vi "MOVE BIAS.vi"(0 "SweepQ in":refnum<queue>, 1 "x":dbl, 2 "return value":cluster{"x":dbl, "y":dbl}, 5 "ScanQ in":refnum<queue>, 7 "Boolean":bool, 11 "error in (no error)":errorcluster, 12 "y":dbl, 13 "Bias in":T1 {"Final Y (m)" format="%.3p"; "Final X (m)" format="%.3p"}) -> (3 "X (m)":sgl, 4 "SweepQ out":refnum<queue>, 6 "ScanQ out":refnum<queue>, 14 "Y (m)":sgl, 15 "error out":errorcluster)   [LabVIEW 2025]
uses:
  STM-Auto-Project/QMH CTLS/Scan_Params (QMH).ctl
  STM-Auto-Project/QMH CTLS/Sweeper.ctl
  Magnetic Drift Correction/Bias Cont QMH.ctl
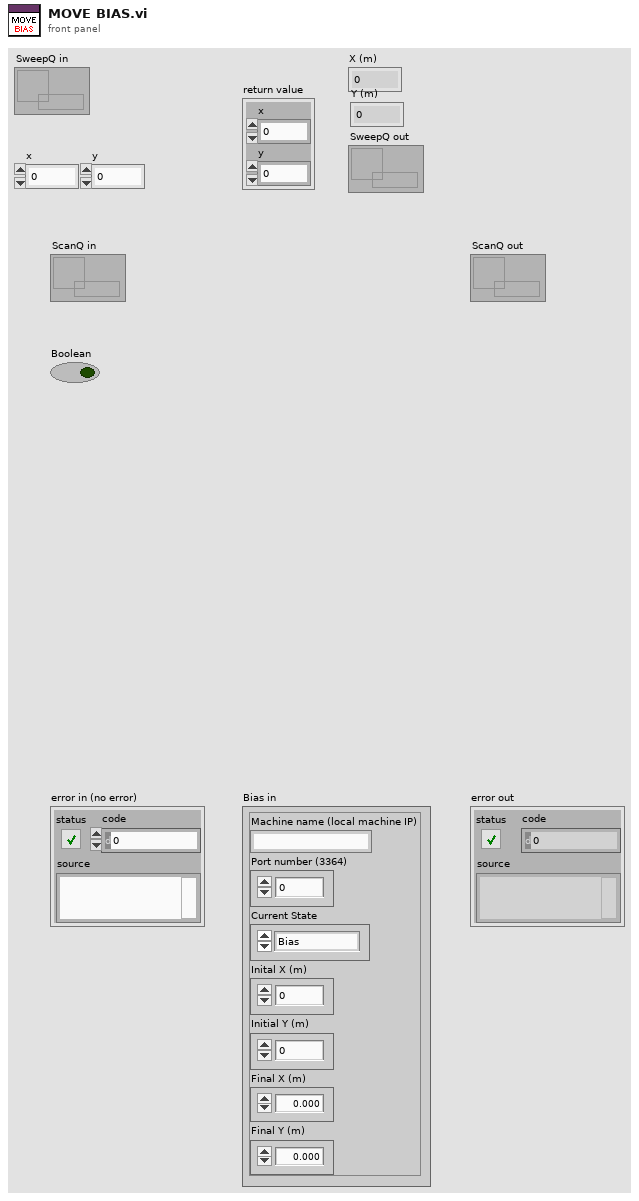
[diagram p1: front panel]
types:
  T1 = typedef "Bias Cont QMH.ctl" = cluster{"Machine name (local machine IP)":string, "Port number (3364)":u32, "Current State":enum16{"Bias", "Stop"}, "Inital X (m)":dbl, "Initial Y (m)":dbl, "Final X (m)":sgl, "Final Y (m)":sgl}
  T2 = enum16{"NO CHANGE", "SET TEMP & FIELD", "SWEEP IDLE", "NEXT TEMP & FIELD", "SWEEP DONE"}
  T3 = typedef "Sweeper.ctl" = cluster{"Temps(K)":dbl[], "Fields(T)":dbl[], "Sweep States":enum16{"NO CHANGE", "SET TEMP & FIELD", "SWEEP IDLE", "NEXT TEMP & FIELD", "SWEEP DONE"}}
  T4 = enum16{"1. BIAS", "2. INIT_SCAN", "3. SCAN_IDLE", "4. INTER_SCAN", "5. NEW_COORDS_&_FRAME", "6. FINAL_SCAN", "7. POLL BIAS ", "8. STOP"}
  T5 = typedef "Scan_Params (QMH).ctl" = cluster{"Setpoint (I)":dbl[], "Bias (V)":dbl[], "Number of scans":u8, "Port number (3364)":u32, "Avoid zero threshold (V)":dbl, "Current State":enum16{"1. BIAS", "2. INIT_SCAN", "3. SCAN_IDLE", "4. INTER_SCAN", "5. NEW_COORDS_&_FRAME", "6. FINAL_SCAN", "7. POLL BIAS ", "8. STOP"}}
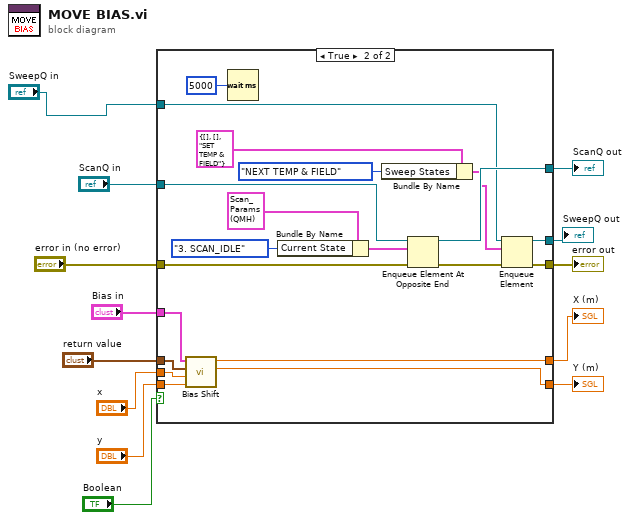
[diagram p0: block diagram]
diagram:
  n1 = case shown="True" "Boolean" {
    tunnel: "return value" -> [_ w29]
    tunnel: "ScanQ in" -> [w17 w33]
    tunnel: [w17 w34] -> w10
    tunnel: [w16 w35] -> w11
    tunnel: "error in (no error)" -> [w16 w31]
    tunnel: [_ w36] -> w2
    tunnel: [w15 w28] -> w6
    tunnel: "Bias in" -> [_ w27]
    tunnel: "SweepQ in" -> [_ w25]
    tunnel: [w14 w24] -> w5
    tunnel: "x" -> [w15 w23]
    tunnel: "y" -> [w14 w22]
    frame False {
    }
    frame True {
      n2 = call "Bias Shift.vi"("y"=w22, "x"=w23, "Translation (m)"=w29, "Bias Controller"=w27) -> ("Y (m)"=w24:sgl, "X (m)"=w28:sgl)  [unwired: 6 in]
      n3 = Wait (ms)(milliseconds to wait=u32 5000) -> ()  [unwired: 1 out]
      n4 = Bundle By Name(cluster=T5 {"Setpoint (I)"=[], "Bias (V)"=[], "Number of scans"=1, "Port number (3364)"=3364, "Avoid zero threshold (V)"=0.004999999888241291, "Current State"=enum."1. BIAS"} ("element"), "Current State"=T4."3. SCAN_IDLE") -> (w26:T5)
      n5 = Bundle By Name(cluster=T3 {"Temps(K)"=[], "Fields(T)"=[], "Sweep States"=enum."SET TEMP & FIELD"} ("Temp and Field Range"), "Sweep States"=T2."NEXT TEMP & FIELD") -> (w18:T3)
      n6 = Enqueue Element At Opposite End(queue=w33, element=w26, error in (no error)=w31) -> (queue out=w34:refnum<queue>, error out=w30:errorcluster)  [unwired: 1 in, 1 out]
      n7 = Enqueue Element(queue=w25, element=w18, error in (no error)=w30) -> (queue out=w36:refnum<queue>, error out=w35:errorcluster)  [unwired: 1 in, 1 out]
    }
  }
  "error out" <- w11
  "ScanQ out" <- w10
  "X (m)" <- w6
  "Y (m)" <- w5
  "SweepQ out" <- w2
